vi "time_logic.vi"(8 "Boolean in":bool, 9 "timout":i32, 10 "Elapsed Time":u32, 11 "Start Time":u32) -> (1 "Boolean out":bool)   [LabVIEW 2015]
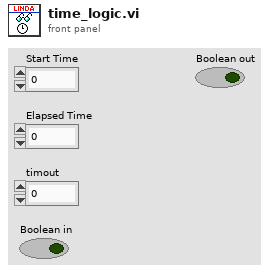
[diagram p1: front panel]
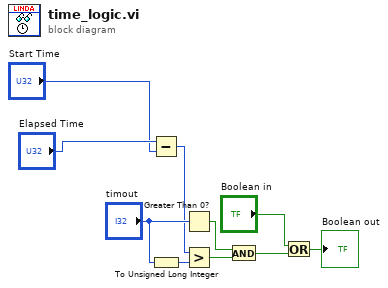
[diagram p0: block diagram]
diagram:
  n1 = Subtract(x="Elapsed Time", y="Start Time") -> (x-y=w4:u32)
  n2 = To Unsigned Long Integer(number="timout") -> (unsigned 32bit integer=w3:u32)
  n3 = Greater Than 0?(x="timout") -> (x > 0?=w7:bool)
  n4 = Greater?(x=w4, y=w3) -> (0:w6:bool)
  n5 = And(x=w7, y=w6) -> (x .and. y?=w8:bool)
  n6 = Or(x="Boolean in", y=w8) -> (x .or. y?=→"Boolean out":bool)
